vi "Add to Msg Chain.vi"(9 "New":string, 10 "Separator (-)":string=" - ", 11 "Msg Chain in":string) -> (2 "Msg Chain out":string)   [LabVIEW 2023, in "UI Interaction.lvclass"]
uses:
  UI Interaction.lvclass
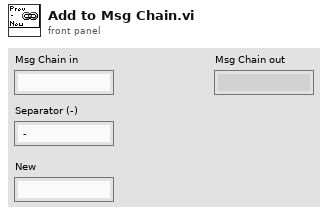
[diagram p1: front panel]
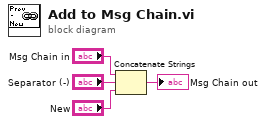
[diagram p0: block diagram]
diagram:
  n1 = Concatenate Strings("Msg Chain in", "Separator (-)", "New") -> (→"Msg Chain out":string)
